vi "array to Logcluster.vi"(0 "UD array":string[](array[string]), 11 "error in (no error)":errorcluster) -> (4 "Log Cluster out":T1, 15 "error out":errorcluster)   [LabVIEW 2012]
uses:
  typedef/Log_User_Data.ctl
  typedef/User Accounts.ctl
  typedef/User_Data_Cluster.ctl
panel:
  in  "Log Cluster":T1
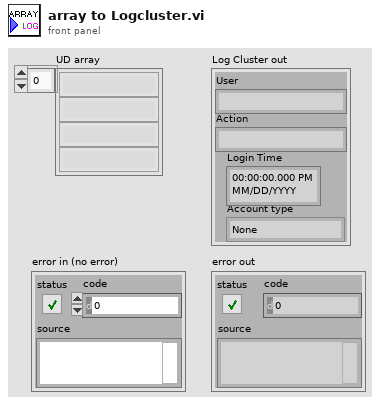
[diagram p1: front panel]
types:
  T1 = typedef "Log_User_Data.ctl" = cluster{"User":string, "Action":string, "Account type":T2, "Login Time ":timestamp}
  T2 = typedef "User Accounts.ctl" = enum16{"None", "User", "Admin"}
  T3 = typedef "User_Data_Cluster.ctl" = cluster{"Usuario":string, "Password":string, "Account type":T2, "Time Stamp":timestamp}
  T4 = cluster{"UD array[0]":string, "UD array[1]":string, "UD array[2]":string, "UD array[3]":string, "UD array[4]":string, "UD array[5]":string, "UD array[6]":string, "UD array[7]":string, "UD array[8]":string}
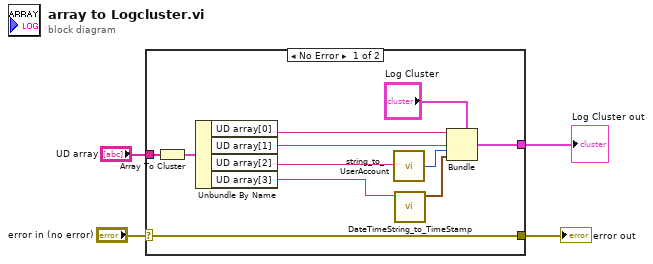
[diagram p0: block diagram]
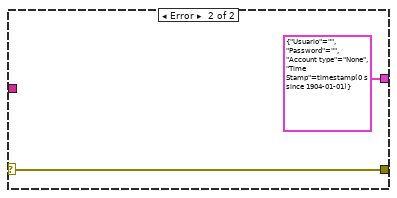
[diagram p2: hidden frame]
diagram:
  n1 = case shown="No Error" "error in (no error)" {
    selector: "error in (no error)" -> [w6 w17]
    tunnel: [w10 T3 {"Usuario"="", "Password"="", "Account type"=enum."None", "Time Stamp"=timestamp(0 s since 1904-01-01)} ("User-data cluster in")] -> w1
    tunnel: "UD array" -> [w9 _]
    tunnel: [w6 w17] -> w2
    frame No Error {
      n2 = Array To Cluster(array=w9) -> (cluster=w8:T4)
      n3 = Unbundle By Name(w8) -> ("UD array[0]"=w12:string, "UD array[1]"=w7:string, "UD array[2]"=w13:string, "UD array[3]"=w15:string)
      n4 = call "string_to_UserAccount.vi"("String account"=w13) -> ("Account"=w11:T2)
      n5 = call "DateTimeString_to_TimeStamp.vi"("%m/%d/%Y %H:%M:%S string"=w15) -> ("Time Stamp"=w14:timestamp)  [unwired: 9 in, 1 out]
      n6 = Bundle(cluster="Log Cluster", "User"=w12, "Action"=w7, "Account type"=w11, "Login Time"=w14) -> (w10:T1)
    }
    frame Error {
    }
  }
  "error out" <- w2
  "Log Cluster out" <- w1
